vi "UseFileImage.vi"(8 "error in (no error)":errorcluster, 10 "File Path":path, 11 "Image Name":string="Source") -> (0 "error out":errorcluster, 3 "Original Image":T1(plugin-control))   [LabVIEW 2017]
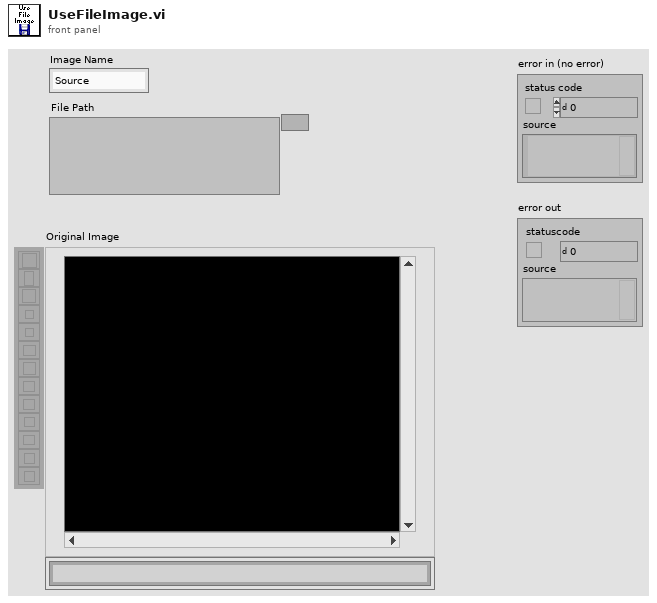
[diagram p1: front panel]
types:
  T1 = typedef "IMAQ Image.ctl" = refnum<image>
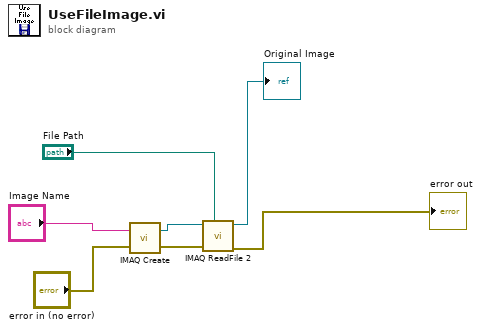
[diagram p0: block diagram]
diagram:
  n1 = call "IMAQ Create"("Image Name"="Image Name", "error in (no error)"="error in (no error)") -> ("New Image"=w5:T1, "error out"=w4:errorcluster)  [unwired: 3 in]
  n2 = call "IMAQ ReadFile 2"("File Path"="File Path", "error in (no error)"=w4, "Image"=w5) -> ("error out"=→"error out":errorcluster, "Image Out"=→"Original Image":T1)  [unwired: 4 in, 3 out]
